vi "Create Path.vi"(7 "Configuration":T1, 8 "error in (no error)":errorcluster) -> (0 "error out":errorcluster, 3 "created path":path)   [LabVIEW 2018]
uses:
  Controls/Path Command.ctl
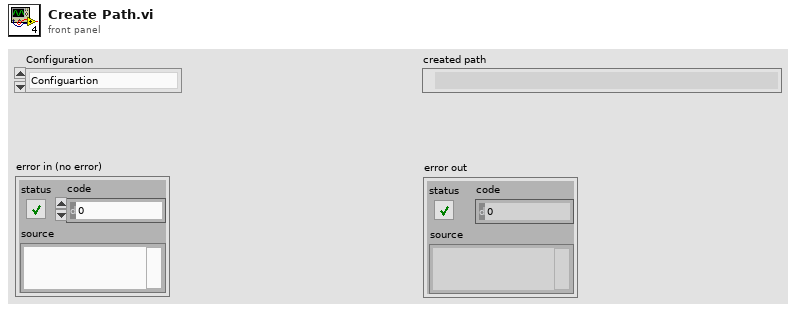
[diagram p1: front panel]
types:
  T1 = typedef "Path Command.ctl" = enum16{"Configuartion"}
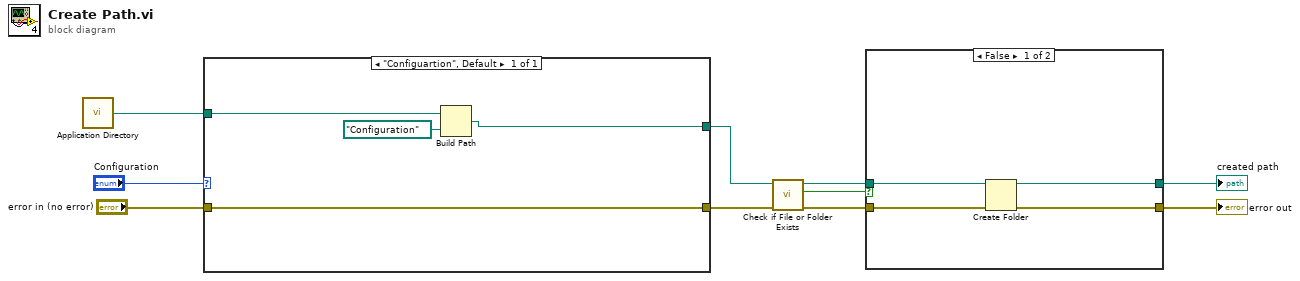
[diagram p0: block diagram]
diagram:
  n1 = call <vilib>:"Application Directory.vi"() -> ("Application Directory"=w9:path)
  n2 = case shown="\"Configuartion\", Default" "Configuration" {
    tunnel: w9 -> [w14]
    tunnel: [w12] -> w8
    tunnel: "error in (no error)" -> [w11]
    tunnel: [w11] -> w4
    frame "Configuartion", Default {
      n3 = Build Path(base path=w14, name or relative path=path "Configuration") -> (appended path=w12:path)
    }
  }
  n4 = call <vilib>:"Check if File or Folder Exists.vi"("error in (no error)"=w4, "path"=w8) -> ("error out"=w3:errorcluster, "file or folder exists?"=w7:bool, "dup path"=w6:path)  [unwired: 7 in]
  n5 = case shown="False" w7 {
    tunnel: w6 -> [w17 w20]
    tunnel: w3 -> [w18 w19]
    tunnel: [w16 w19] -> w2
    tunnel: [w15 w20] -> w1
    frame False {
      n6 = Create Folder(path (use dialog)=w17, error in=w18) -> (created path=w15:path, error out=w16:errorcluster)  [unwired: 1 in, 1 out]
    }
    frame True {
    }
  }
  "error out" <- w2
  "created path" <- w1
